vi "UI-Cmd-Init.vi"(9 "Data":variant, 10 "Queue":refnum<queue>, 11 "UI State In":T1) -> (0 "error out":errorcluster, 3 "UI State Out":T1)   [LabVIEW 2024, in "CustomActions.lvlib"]
uses:
  CustomActions.lvlib
  UI-State--cluster.ctl
  UI-Refs--cluster.ctl
  UI-Platform--radio.ctl
  UI-ErrorCheckingLevel--radio.ctl
  UI-Cmd--cluster.ctl
  UI-Cmd--enum.ctl
  57d78318-9664-4939-99cb-6267cdd54025.vi
  <vilib>/Utility/error.llb/Error Cluster From Error Code.vi
  <vilib>/ErrorRing/Error Ring.xnode
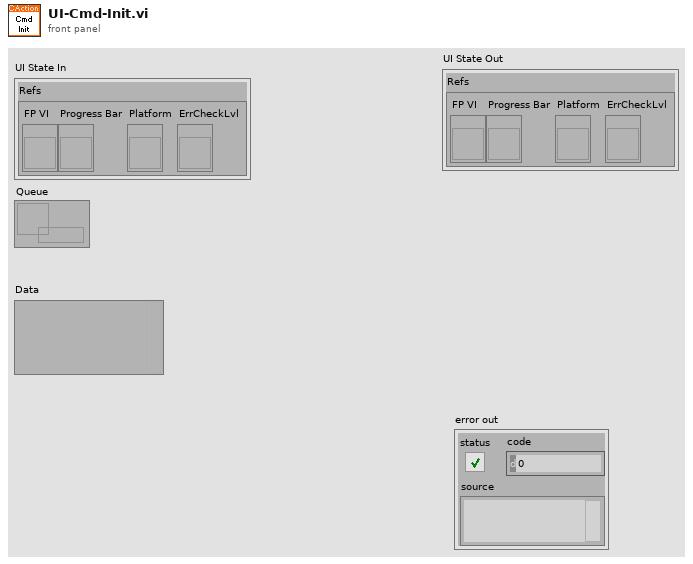
[diagram p1: front panel]
types:
  T1 = typedef "CustomActions.lvlib/UI-State--cluster.ctl" = cluster{"Refs":T2}
  T2 = typedef "CustomActions.lvlib/UI-Refs--cluster.ctl" = cluster{"FP VI":refnum<vi>, "Progress Bar":refnum<vi>, "Platform":refnum<vi>, "ErrCheckLvl":refnum<vi>}
  T3 = enum16{"Init FP Window", "Init Progress Bar", "Init Platform Radio", "Init ErrCheckLvl"}
  T4 = enum16{"Init FP Window", "Init Progress Bar", "Init Platform Radio", "Init ErrCheckLvl"}[]
  T5 = typedef "CustomActions.lvlib/UI-Platform--radio.ctl" = enum32{"Windows 32 Bit", "Windows 64 Bit", "Linux"}
  T6 = typedef "CustomActions.lvlib/UI-ErrorCheckingLevel--radio.ctl" = enum32{"Maximum", "Default", "Disabled"}
  T7 = typedef "CustomActions.lvlib/PlatformType--enum.ctl" = enum16{"Unknown", "Win32", "Win64", "Linux64"}
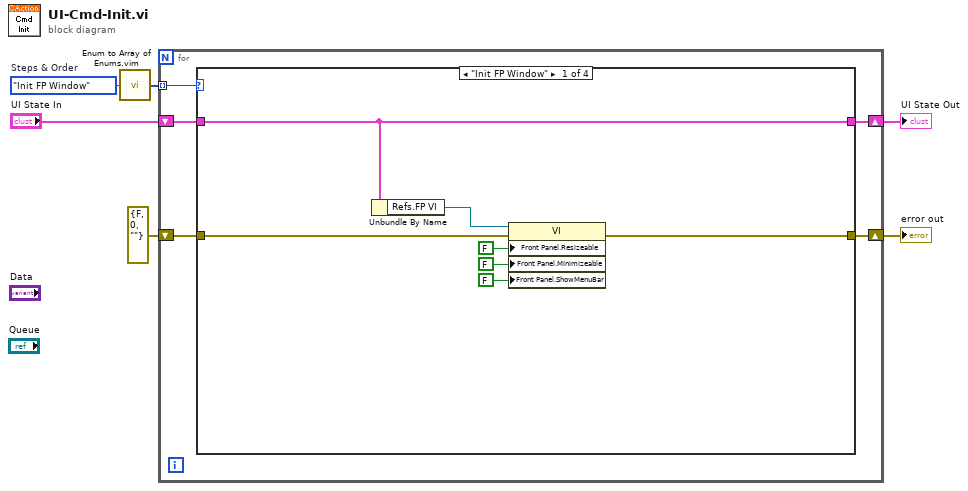
[diagram p0: block diagram]
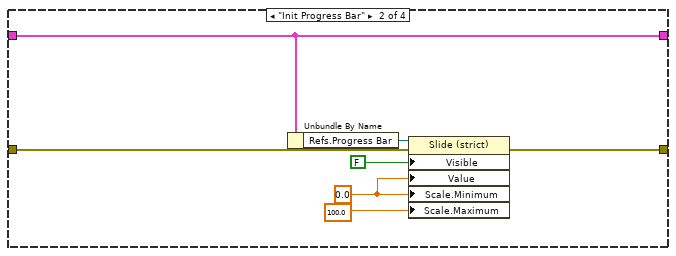
[diagram p2: hidden frame]
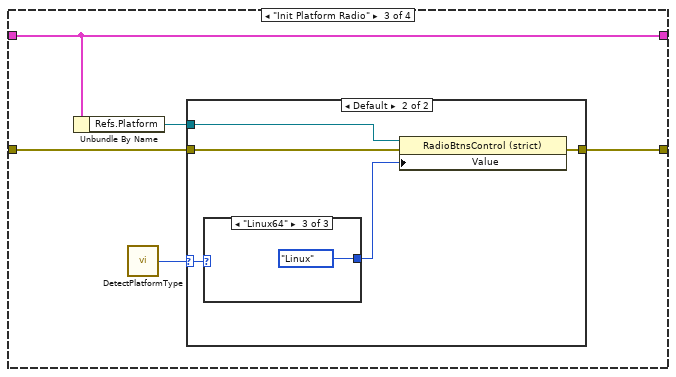
[diagram p3: hidden frame]
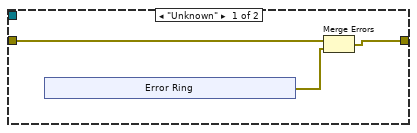
[diagram p4: hidden frame]
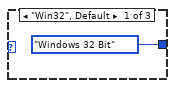
[diagram p5: hidden frame]
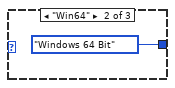
[diagram p6: hidden frame]
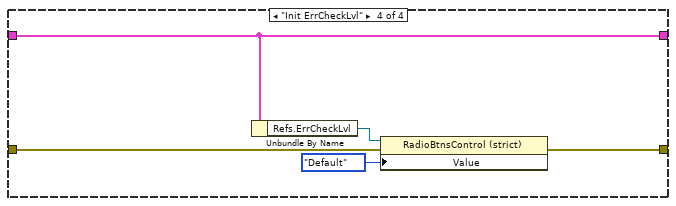
[diagram p7: hidden frame]
diagram:
  w3 = T3."Init FP Window"  # Steps & Order
  n1 = call "Enum to Array of Enums.vim"("enum"=w3) -> ("array of enums"=w2:T4)
  n2 = for {
    shift-right: [w9] -> w4
    shift-left: "UI State In" -> [w11]
    tunnel: w2 -> [w8] mode=indexing
    shift-right: [w10] -> w5
    shift-left: errorcluster {"status"=FALSE, "code"=0, "source"=""} ("error out") -> [w7]
    n3 = case shown="\"Init FP Window\"" w8 {
      tunnel: w11 -> [w16 w21 w28 w47]
      tunnel: [w17 w19 w27 w48] -> w10
      tunnel: [w16 w21 w28 w47] -> w9
      tunnel: w7 -> [w18 w20 w26 w46]
      frame "Init FP Window" {
        n4 = Unbundle By Name(w16) -> ("Refs.FP VI"=w15:refnum<vi>)
        n5 = property class="VI"(reference=w15, error in=w18, "Front Panel.Resizeable"=FALSE ("Front Panel Window:Resizable"), "Front Panel.Minimizeable"=FALSE ("Front Panel Window:Minimizable"), "Front Panel.ShowMenuBar"=FALSE ("Front Panel Window:Show Menu Bar")) -> (error out=w17:errorcluster)  [unwired: 1 out]
      }
      frame "Init Progress Bar" {
        w23 = 0.0 ("Scale.Range:Minimum")
        n6 = Unbundle By Name(w21) -> ("Refs.Progress Bar"=w25:refnum<vi>)
        n7 = property class="Slide (strict)"(reference=w25, error in=w20, "Visible"=FALSE, "Value"=w23, "Scale.Minimum"=w23, "Scale.Maximum"=100.0 ("Scale.Range:Maximum")) -> (error out=w19:errorcluster)  [unwired: 1 out]
      }
      frame "Init Platform Radio" {
        n8 = Unbundle By Name(w28) -> ("Refs.Platform"=w30:refnum<vi>)
        n9 = call "DetectPlatformType.vi"() -> ("Platform Type"=w29:T7)
        n10 = case shown="Default" w29 {
          selector: w29 -> [_ w38]
          tunnel: w26 -> [w33 w42]
          tunnel: [w32 w41] -> w27
          tunnel: w30 -> [_ w40]
          frame "Unknown" {
            n11 = xnode "Error Ring"() -> ("error out"=w31:errorcluster)
            n12 = Merge Errors(w33, w31) -> (w32:errorcluster)
          }
          frame Default {
            n13 = case shown="\"Linux64\"" w38 {
              tunnel: [UI-Platform--radio."Windows 32 Bit" ("Value") UI-Platform--radio."Windows 64 Bit" ("Value") UI-Platform--radio."Linux" ("Value")] -> w39
              frame "Win32", Default {
              }
              frame "Win64" {
              }
              frame "Linux64" {
              }
            }
            n14 = property class="RadioBtnsControl (strict)"(reference=w40, error in=w42, "Value"=w39) -> (error out=w41:errorcluster)  [unwired: 1 out]
          }
        }
      }
      frame "Init ErrCheckLvl" {
        n15 = Unbundle By Name(w47) -> ("Refs.ErrCheckLvl"=w50:refnum<vi>)
        n16 = property class="RadioBtnsControl (strict)"(reference=w50, error in=w46, "Value"=UI-ErrorCheckingLevel--radio."Default") -> (error out=w48:errorcluster)  [unwired: 1 out]
      }
    }
  }
  "UI State Out" <- w4
  "error out" <- w5
